vi "Photon Counter Control Panel (No Objects).vi"(8 "error in (no error)":errorcluster) -> (0 "error out":errorcluster)   [LabVIEW 2012]
uses:
  SR400/Public/Typedefs.llb/Gate Mode.ctl
  SR400/SR400.lvlib
panel:
  in  "VISA Resource Name":refnum<visa-resource-name>="GPIB0::23::INSTR"
  in  "Photon Counter SR 400":T1={"Mode"=0, "Count Time"=0.0, "Trigger Frequency"=10000000.0, "Trigger External?"=FALSE, "Gate A Mode"=0, "Gate A Width"=0.0, "Gate A Delay"=0.0, "Gate B Mode"=0, "Gate B Width"=0.0, "Gate B Delay"=0.0} {"Mode" items=["A,B For T Preset", "A-B For T Preset", "A+B For T Preset", "A For B Preset"]; "Gate A Mode" items=["CW", "Fixed"]; "Gate B Mode" items=["CW", "Fixed"]}
  out "Update visible/hidden":bool
  out "Gate B Mode":T2
  out "Gate A Mode":T2
  in  "stop":bool
  in  "Read to Control":bool
  in  "Read":bool
  in  "Initialize":bool
  out "Gate A % Current":dbl
  out "Gate B % Current":dbl
  in  "Gate B % Set":dbl
  in  "Gate A % Set":dbl
  in  "Gate Width: Time / Percent":bool caption="Gate Width\n        Time / Percent"
  in  "Gate Delay Reference\n        Start / Middle":bool
  in  "Gate B Mode Set":T2
  in  "Gate A Mode Set":T2
  out "Trigger Freq Current":dbl[unit]=42077.399999999994 caption="Trigger Freq"
  in  "Trigger Freq Set":dbl[unit]=42077.399999999994 caption="Trigger Freq."
  in  "Set Time & Freq.":bool
  in  "# Triggers vs Freq/Time":bool
  out "# of Cycles Current":dbl format="%^#_6g"
  in  "# of Cycles Set":dbl format="%^#_6g"
  in  "Set # of Triggers":bool
  in  "Internal / External":bool
  out "cpsB":dbl[unit] caption="CPS B"
  out "cpsA":dbl[unit] caption="CPS A"
  in  "Gate B Width Set":dbl[unit] caption="Gate B Width"
  in  "Gate A Width Set":dbl[unit]
  out "Gate A Width":dbl[unit] format="%^#_6g"
  out "Gate B Width":dbl[unit] format="%^#_6g"
  out "Gate B Delay":dbl[unit]
  out "Gate A Delay":dbl[unit]
  in  "Gate B Delay Set":dbl[unit]
  in  "Gate A Delay Set":dbl[unit]
  in  "Set Gate Delays":bool
  in  "Set Gate Mode":bool
  in  "Set Gate Widths":bool
  in  "Read Channels":bool
  in  "Count Time Set":dbl[unit]
  out "Count Time Current":dbl[unit]=1.0 min=0.0 max=10000.0 step=1.0 format="%#_7g"
  in  "Set Count Time":bool
  # "Gates"
  # "Trigger"
  # "Gate A"
  # "Gate B"
  # "Channels"
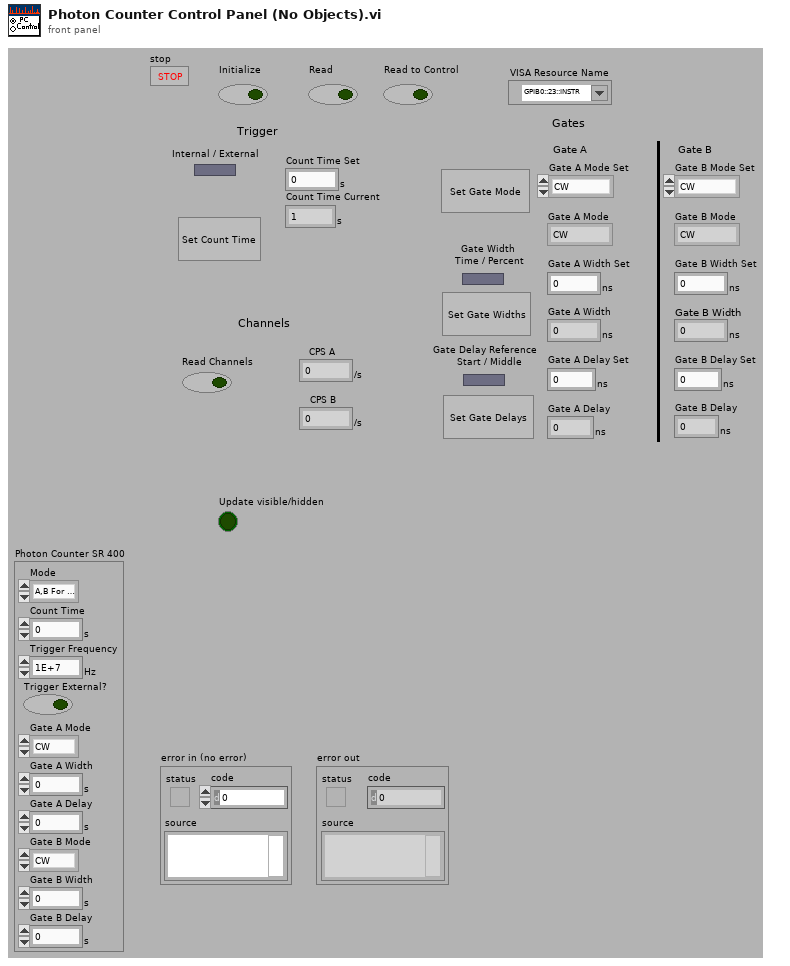
[diagram p1: front panel]
types:
  T1 = cluster{"Mode":u16, "Count Time":dbl[unit], "Trigger Frequency":dbl[unit], "Trigger External?":bool, "Gate A Mode":u16, "Gate A Width":dbl[unit], "Gate A Delay":dbl[unit], "Gate B Mode":u16, "Gate B Width":dbl[unit], "Gate B Delay":dbl[unit]}
  T2 = typedef "SR400.lvlib/Gate Mode.ctl" = enum16{"CW", "Fixed", "Scan"}
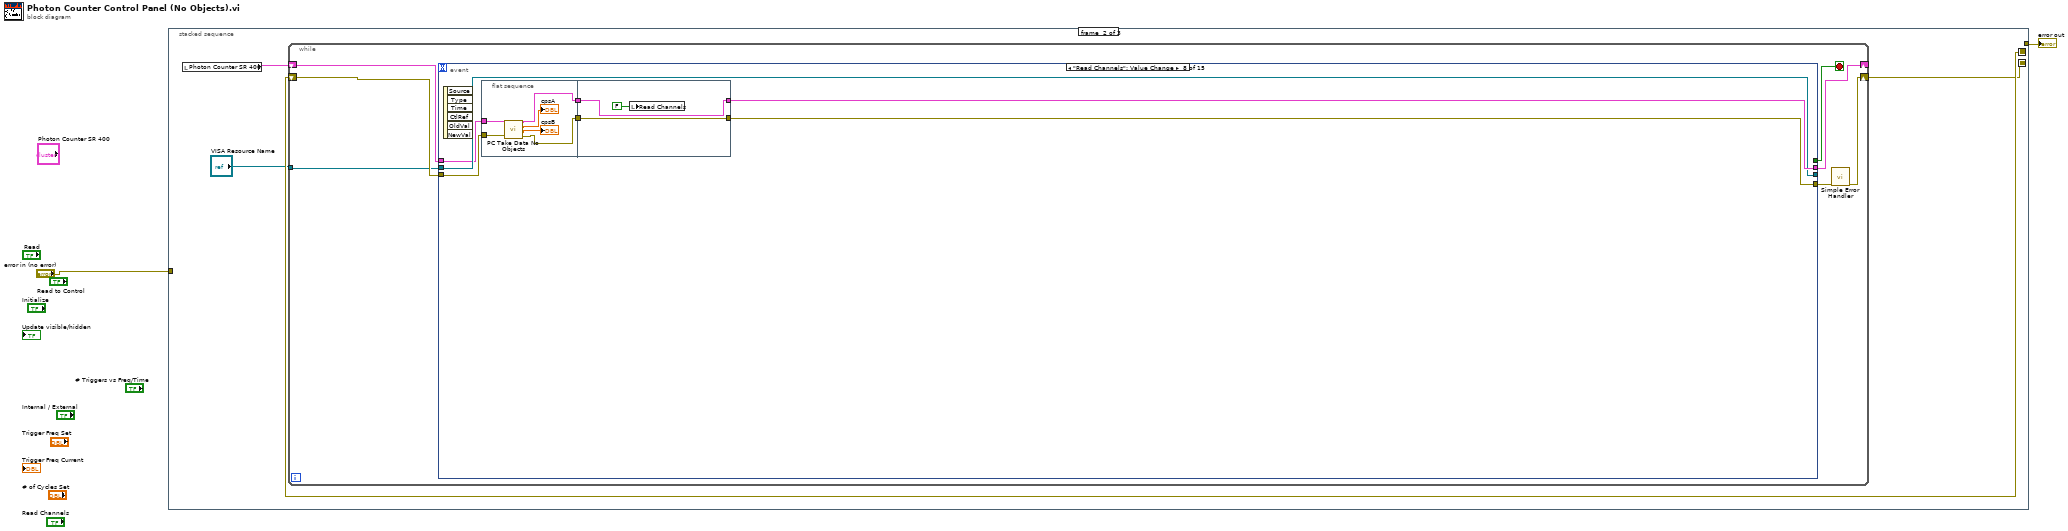
[diagram p0: block diagram]
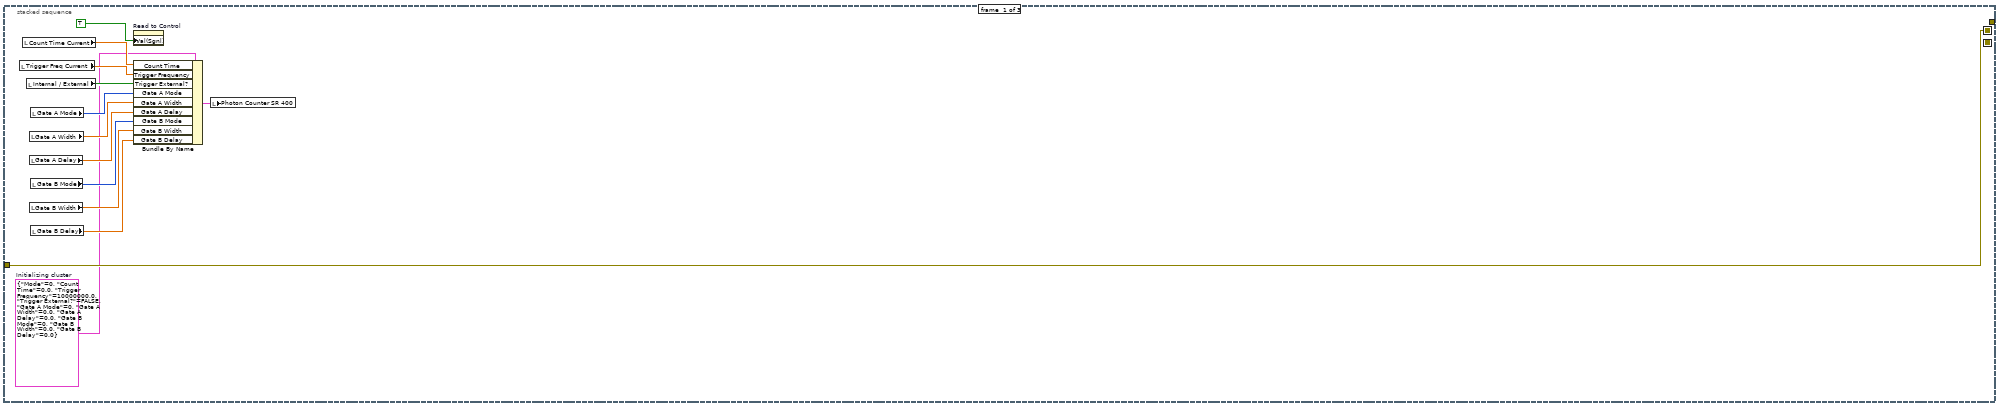
[diagram p2: hidden frame]
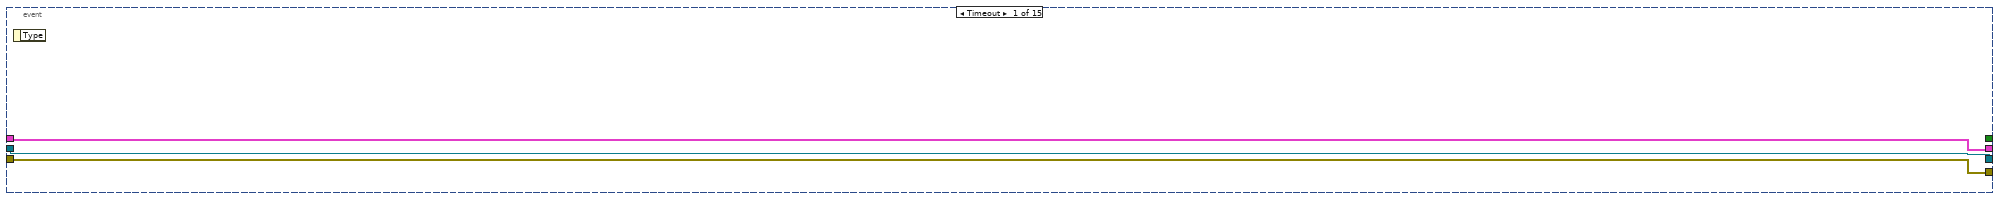
[diagram p3: hidden frame]
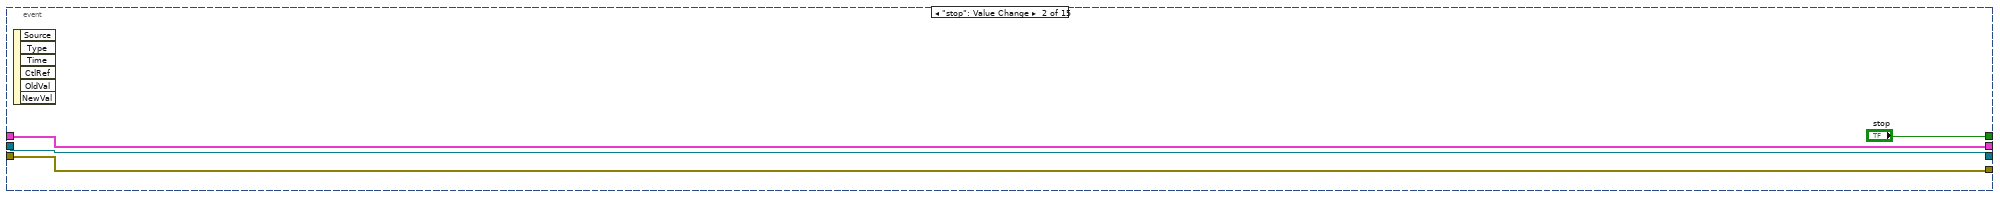
[diagram p4: hidden frame]
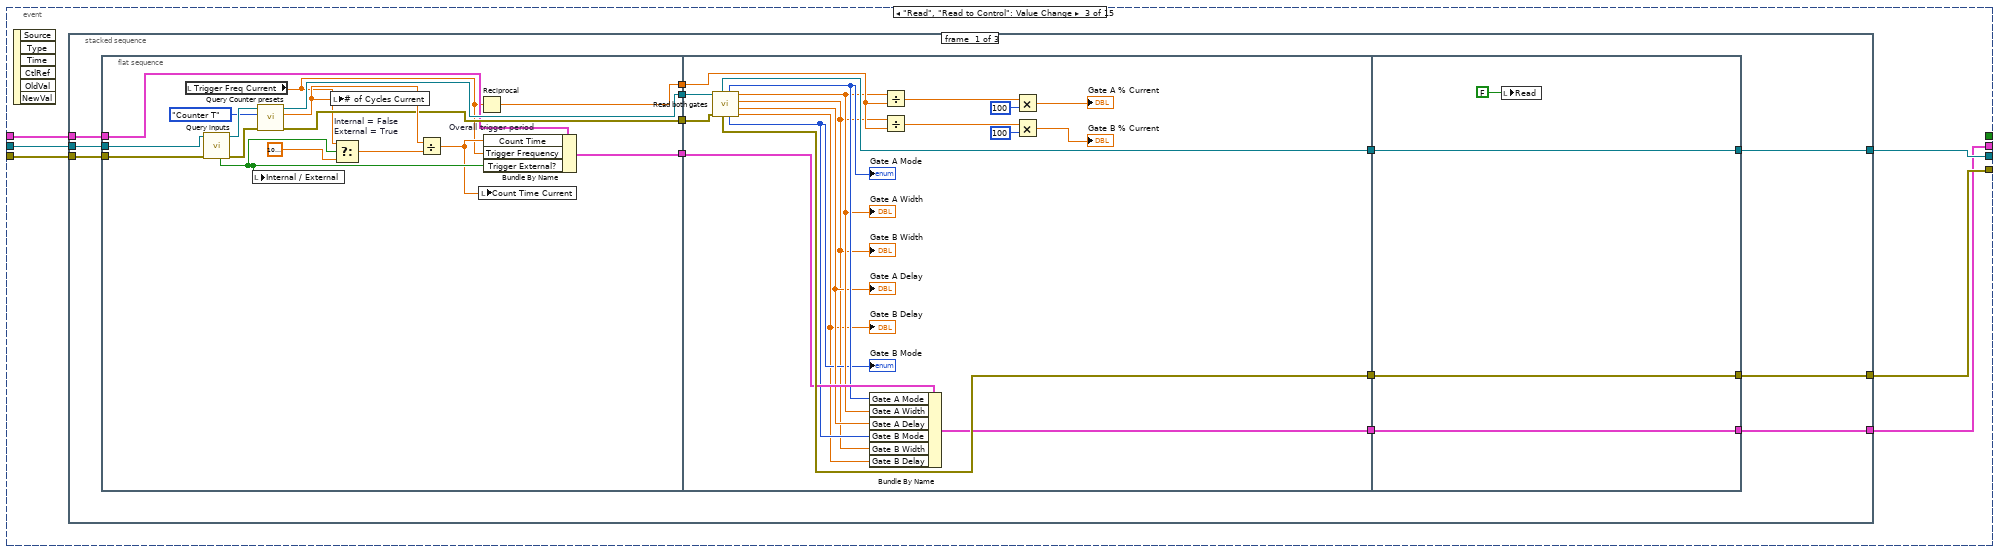
[diagram p5: hidden frame]
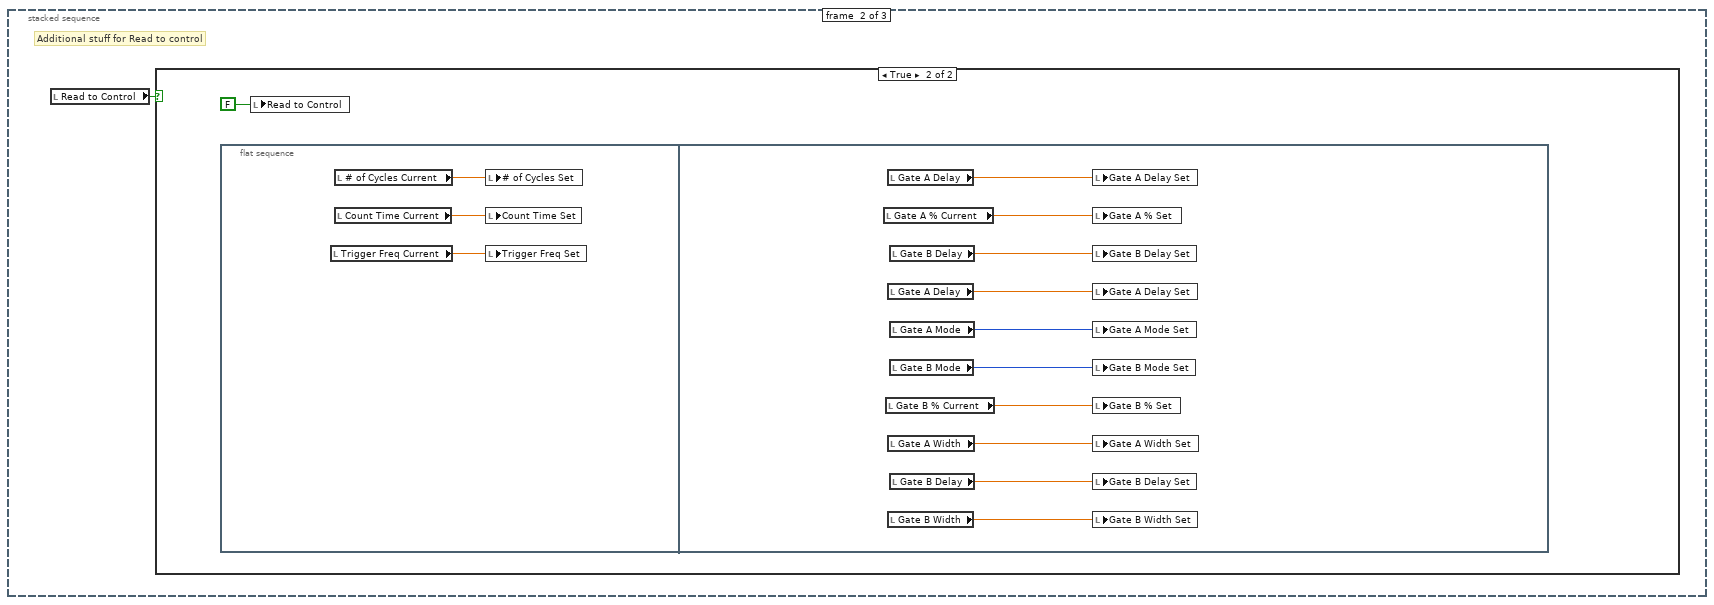
[diagram p6: hidden frame]
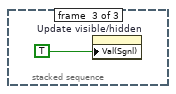
[diagram p8: hidden frame]
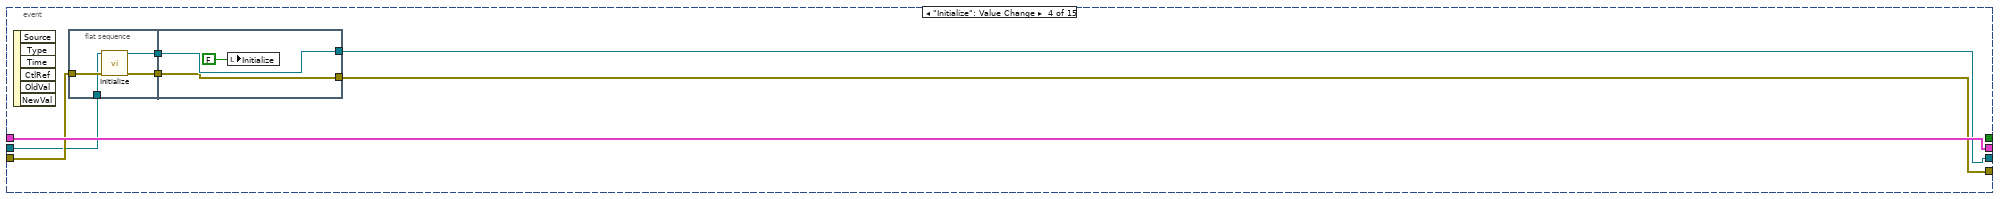
[diagram p9: hidden frame]
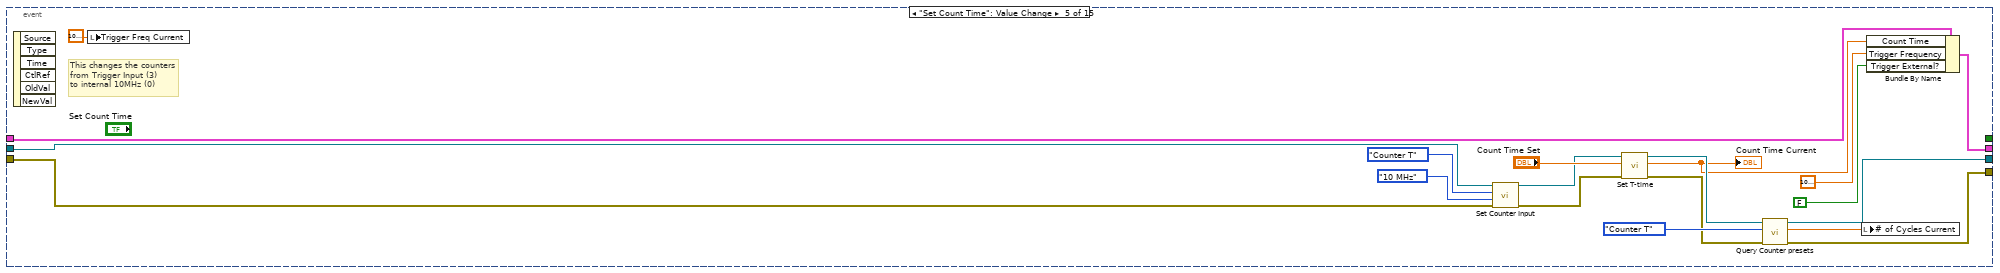
[diagram p10: hidden frame]
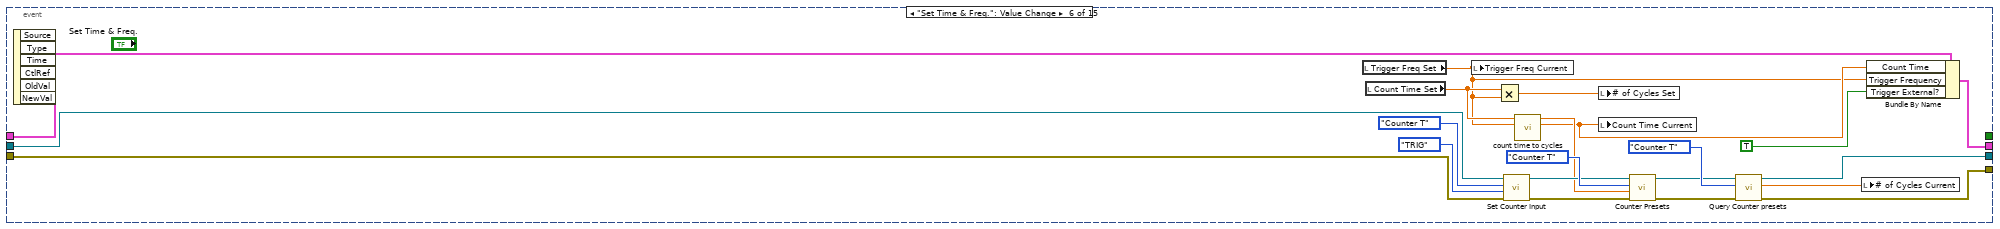
[diagram p11: hidden frame]
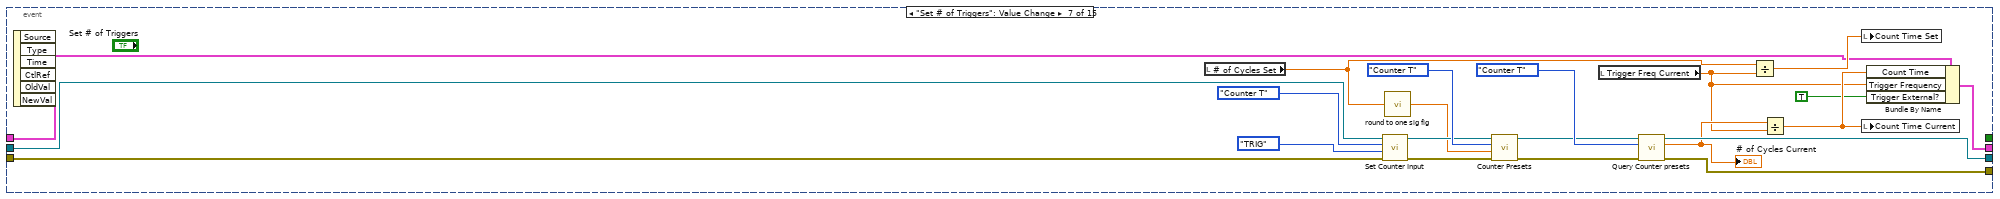
[diagram p12: hidden frame]
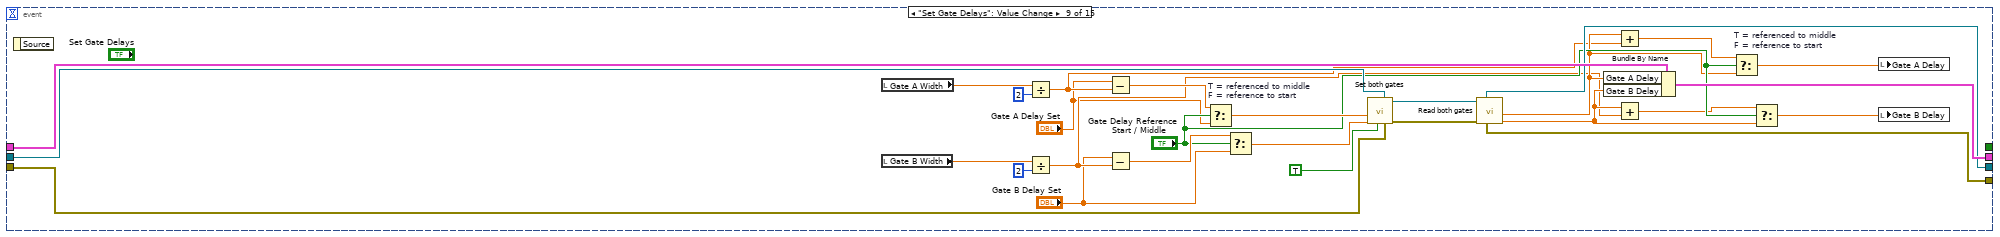
[diagram p13: hidden frame]
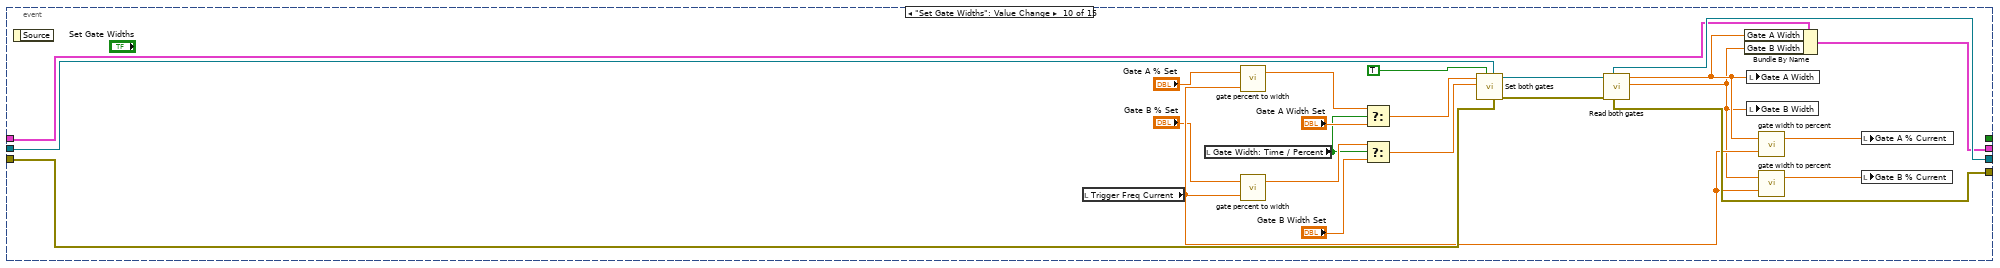
[diagram p14: hidden frame]
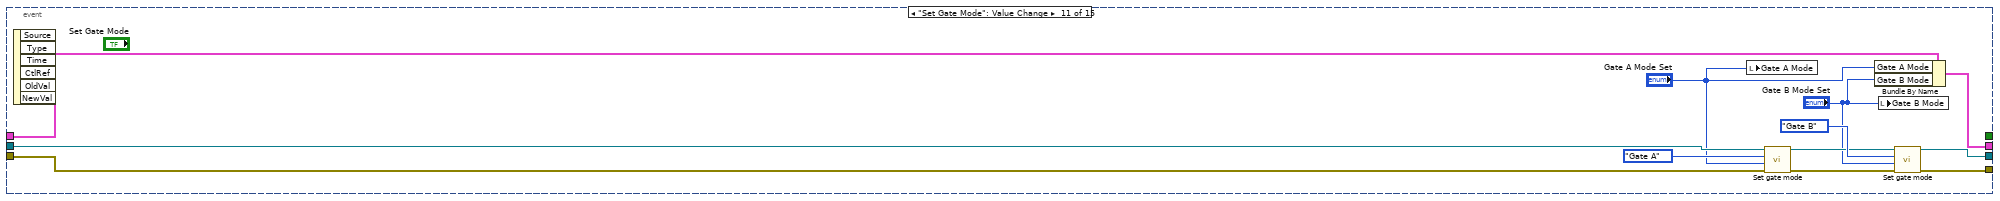
[diagram p15: hidden frame]
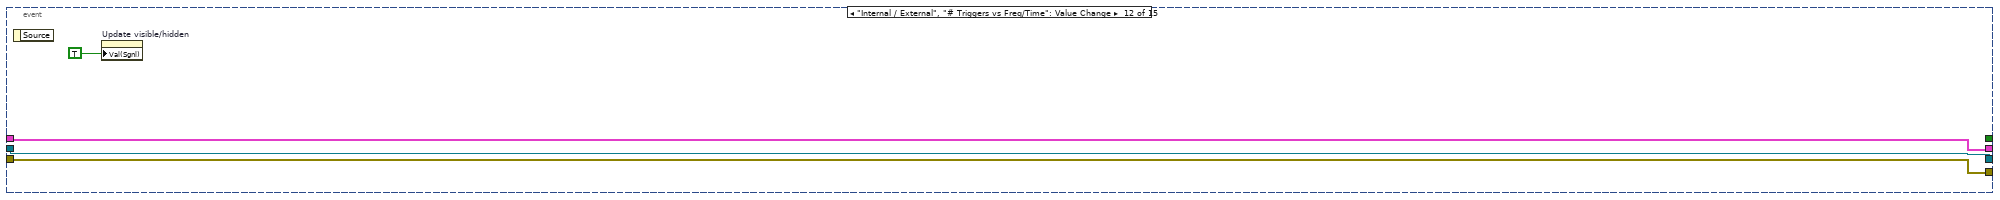
[diagram p16: hidden frame]
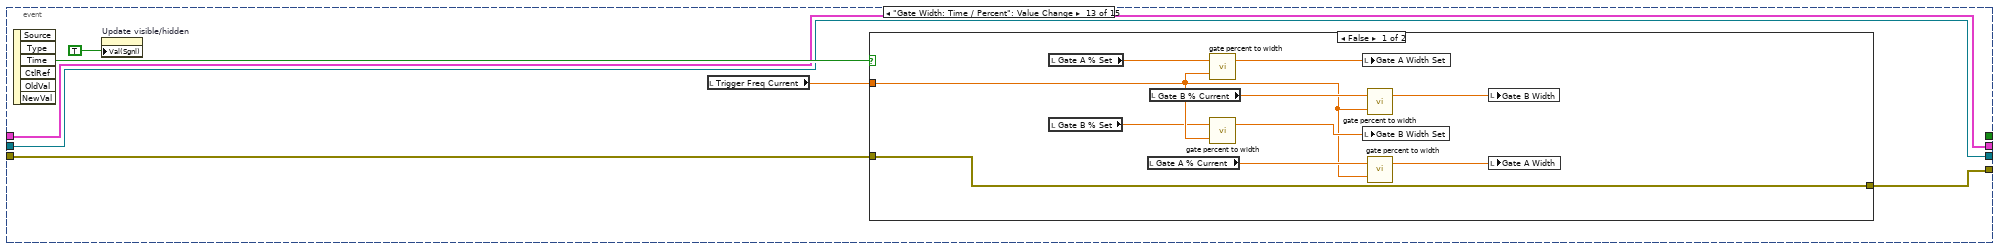
[diagram p17: hidden frame]
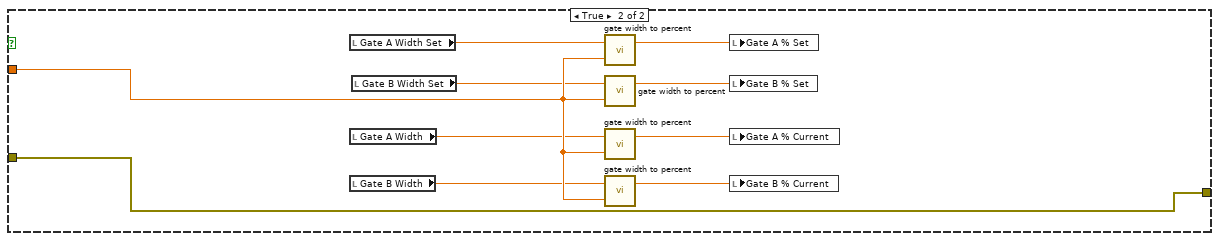
[diagram p18: hidden frame]
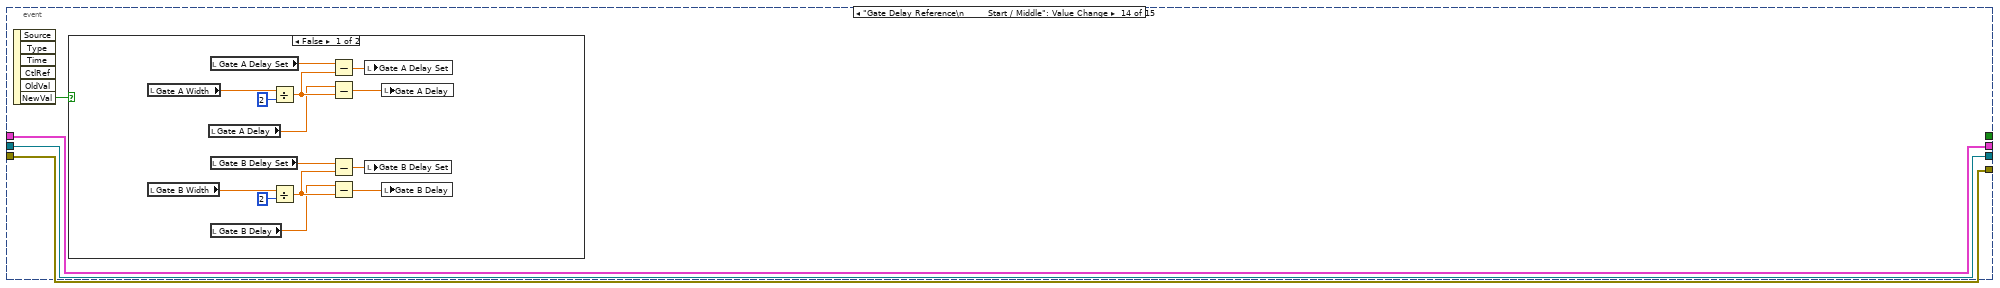
[diagram p19: hidden frame]
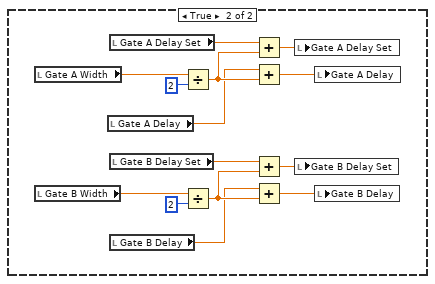
[diagram p20: hidden frame]
diagram:
  n1 = stacked-sequence {
    seq-local: [w5 _ _] -> [_ w19 _]
    seq-local: [_ w18 _] -> [_ _ w338]
    tunnel: "error in (no error)" -> [w5 _ _]
    tunnel: [_ _ w338] -> w2
    frame #0 {
      w3 = T1 {"Mode"=0, "Count Time"=0.0, "Trigger Frequency"=10000000.0, "Trigger External?"=FALSE, "Gate A Mode"=0, "Gate A Width"=0.0, "Gate A Delay"=0.0, "Gate B Mode"=0, "Gate B Width"=0.0, "Gate B Delay"=0.0}  # Initializing cluster
      n2 = local read "Trigger Freq Current"() -> (w13:dbl[unit])
      n3 = local read "Count Time Current"() -> (w14:dbl[unit])
      n4 = local read "Internal / External"() -> (w12:bool)
      n5 = local read "Gate A Width"() -> (w10:dbl[unit])
      n6 = local read "Gate A Delay"() -> (w9:dbl[unit])
      n7 = local read "Gate B Width"() -> (w7:dbl[unit])
      n8 = local read "Gate A Mode"() -> (w11:T2)
      n9 = local read "Gate B Mode"() -> (w6:T2)
      n10 = local read "Gate B Delay"() -> (w8:dbl[unit])
      n11 = property on="Read to Control" class="Bool (strict)"("Val(Sgnl)"=TRUE ("Value (Signaling)")) -> ()  [unwired: 2 in, 2 out]
      n12 = Bundle By Name(cluster=w3, "Count Time"=w14, "Trigger Frequency"=w13, "Trigger External?"=w12, "Gate A Mode"=w11, "Gate A Width"=w10, "Gate A Delay"=w9, "Gate B Mode"=w6, "Gate B Width"=w7, "Gate B Delay"=w8) -> (w4:T1)
      n13 = local write "Photon Counter SR 400"(w4) -> ()
    }
    frame #1 {
      n14 = local read "Photon Counter SR 400"() -> (w17:T1)
      n15 = while {
        shift-right: [w22] -> _
        shift-left: w17 -> [w21]
        shift-right: [w25] -> w18
        shift-left: w19 -> [w23]
        tunnel: "VISA Resource Name" -> [w20]
        stop <- w24 stop-if-true
        n16 = event shown="[7] \"Read Channels\": Value Change" {
          selector: _ -> [_ _ _ _ _ _ _ _ _ _ _ _ _ _ _]
          dyn-events: _ -> [_ _ _ _ _ _ _ _ _ _ _ _ _ _ _]
          timeout: _ -> [_ _ _ _ _ _ _ _ _ _ _ _ _ _ _]
          tunnel: [w28 w31 w37 w108 w137 w156 w180 w186 w212 w244 w254 w265 w268 w294 w327] -> _
          tunnel: w23 -> [w27 w30 w39 w113 w128 w150 w172 w189 w226 w245 w258 w264 w266 w293 w326]
          tunnel: [w27 w30 w36 w112 w136 w157 w179 w188 w210 w243 w255 w264 w267 w293 w326] -> w26
          tunnel: w20 -> [w28 w31 w38 w109 w129 w151 w173 w186 w225 w246 w259 w265 w268 w294 w327]
          tunnel: w21 -> [w29 w32 w35 w114 w126 w145 w166 w185 w224 w230 w253 w263 w269 w295 w325]
          tunnel: [w29 w32 w34 w114 w125 w144 w165 w187 w223 w229 w252 w263 w269 w295 w325] -> w22
          tunnel: [_ "stop" _ _ _ _ _ _ _ _ _ _ _ _ _] -> w24
          event Timeout {
            n17 = event-data() -> ()  [unwired: 2 out]
          }
          event "stop": Value Change {
            n18 = event-data() -> ()  [unwired: 7 out]
          }
          event "Read", "Read to Control": Value Change {
            n19 = event-data() -> ()  [unwired: 7 out]
            n20 = stacked-sequence {
              tunnel: w39 -> [w51 _ _]
              tunnel: w38 -> [w52 _ _]
              tunnel: [w47 _ _] -> w37
              tunnel: [w45 _ _] -> w36
              tunnel: w35 -> [w43 _ _]
              tunnel: [w41 _ _] -> w34
              frame #0 {
                n21 = flat-sequence {
                  tunnel: w52 -> [w68]
                  tunnel: w51 -> [w65]
                  tunnel: [w61] -> w50
                  tunnel: [w60] -> w49
                  tunnel: [w59] -> w48
                  tunnel: w43 -> [w57]
                  tunnel: [w53] -> w42
                  tunnel: w50 -> [w81]
                  tunnel: w49 -> [w80]
                  tunnel: w48 -> [w79]
                  tunnel: [w78] -> w46
                  tunnel: [w77] -> w44
                  tunnel: w42 -> [w76]
                  tunnel: [w69] -> w40
                  tunnel: [w90] -> w47
                  tunnel: w46 -> [w90]
                  tunnel: [w89] -> w45
                  tunnel: w44 -> [w89]
                  tunnel: [w88] -> w41
                  tunnel: w40 -> [w88]
                  frame #0 {
                    n22 = local read "Trigger Freq Current"() -> (w54:dbl[unit])
                    n23 = call "Query inputs.vi"("error in (no error)"=w65, "VISA resource name"=w68) -> ("error out"=w66:errorcluster, "VISA resource name out"=w67:refnum<visa-resource-name>, "Externally-triggered?"=w56:bool)  [unwired: 7 out]
                    n24 = local write "Internal / External"(w56) -> ()
                    n25 = call "Query Counter presets.vi"("error in (no error)"=w66, "Counter (Def: T)"=enum16{"Invalid", "Counter B", "Counter T"}."Counter T" ("i (0)"), "VISA resource name"=w67) -> ("error out"=w60:errorcluster, "Number of triggers"=w62:dbl, "VISA resource name out"=w61:refnum<visa-resource-name>)  [unwired: 6 out]
                    n26 = local write "# of Cycles Current"(w62) -> ()
                    n27 = Select "Internal = False\nExternal = True"(t=w54, s=w56, f=dbl[unit] 10000000.0 ("freq")) -> (s? t:f=w63:dbl[unit])
                    n28 = Divide(x=w62, y=w63) -> (x/y=w55:dbl[unit])
                    n29 = Reciprocal "Overall trigger period"(x=w54) -> (1/x=w59:dbl[unit])
                    n30 = local write "Count Time Current"(w55) -> ()
                    n31 = Bundle By Name(cluster=w57, "Count Time"=w55, "Trigger Frequency"=w54, "Trigger External?"=w56) -> (w53:T1)
                  }
                  frame #1 {
                    n32 = call "Read both gates.vi"("error in (no error)"=w80, "VISA resource name"=w81) -> ("Gate B Delay"=w70:dbl[unit], "Gate A Delay"=w73:dbl[unit], "Gate B Width"=w71:dbl[unit], "Gate A Width"=w74:dbl[unit], "Current mode B"=w72:enum16{"CW", "Fixed", "Scan"}, "Current mode A"=w75:enum16{"CW", "Fixed", "Scan"}, "error out"=w77:errorcluster, "VISA resource name out"=w78:refnum<visa-resource-name>)  [unwired: 2 out]
                    "Gate B Width" <- w71
                    "Gate A Width" <- w74
                    "Gate A Delay" <- w73
                    "Gate B Delay" <- w70
                    "Gate A Mode" <- w75
                    "Gate B Mode" <- w72
                    n33 = Bundle By Name(cluster=w76, "Gate A Mode"=w75, "Gate A Width"=w74, "Gate A Delay"=w73, "Gate B Mode"=w72, "Gate B Width"=w71, "Gate B Delay"=w70) -> (w69:T1)
                    n34 = Divide(x=w74, y=w79) -> (x/y=w83:dbl)
                    n35 = Divide(x=w71, y=w79) -> (x/y=w85:dbl)
                    n36 = Multiply(x=w83, y=i8 100) -> (x*y=→"Gate A % Current":dbl)
                    n37 = Multiply(x=w85, y=i8 100) -> (x*y=→"Gate B % Current":dbl)
                  }
                  frame #2 {
                    n38 = local write "Read"(FALSE ("Read")) -> ()
                  }
                }
              }
              frame #1 {
                # "Additional stuff for Read to control"
                n39 = local read "Read to Control"() -> (w92:bool)
                n40 = case shown="True" w92 {
                  frame False {
                  }
                  frame True {
                    n41 = flat-sequence {
                      frame #0 {
                        n42 = local read "Trigger Freq Current"() -> (w94:dbl[unit])
                        n43 = local read "# of Cycles Current"() -> (w95:dbl)
                        n44 = local read "Count Time Current"() -> (w96:dbl[unit])
                        n45 = local write "# of Cycles Set"(w95) -> ()
                        n46 = local write "Count Time Set"(w96) -> ()
                        n47 = local write "Trigger Freq Set"(w94) -> ()
                      }
                      frame #1 {
                        n48 = local read "Gate A % Current"() -> (w103:dbl)
                        n49 = local read "Gate B % Current"() -> (w105:dbl)
                        n50 = local read "Gate A Delay"() -> (w98:dbl[unit])
                        n51 = local read "Gate A Delay"() -> (w104:dbl[unit])
                        n52 = local read "Gate A Width"() -> (w102:dbl[unit])
                        n53 = local read "Gate B Width"() -> (w97:dbl[unit])
                        n54 = local read "Gate B Delay"() -> (w99:dbl[unit])
                        n55 = local read "Gate A Mode"() -> (w100:T2)
                        n56 = local read "Gate B Mode"() -> (w101:T2)
                        n57 = local read "Gate B Delay"() -> (w106:dbl[unit])
                        n58 = local write "Gate A Delay Set"(w98) -> ()
                        n59 = local write "Gate A % Set"(w103) -> ()
                        n60 = local write "Gate B Delay Set"(w99) -> ()
                        n61 = local write "Gate A Delay Set"(w104) -> ()
                        n62 = local write "Gate A Mode Set"(w100) -> ()
                        n63 = local write "Gate B Mode Set"(w101) -> ()
                        n64 = local write "Gate B % Set"(w105) -> ()
                        n65 = local write "Gate A Width Set"(w102) -> ()
                        n66 = local write "Gate B Delay Set"(w106) -> ()
                        n67 = local write "Gate B Width Set"(w97) -> ()
                      }
                    }
                    n68 = local write "Read to Control"(FALSE ("Read to Control")) -> ()
                  }
                }
              }
              frame #2 {
                n69 = property on="Update visible/hidden" class="Bool (strict)"("Val(Sgnl)"=TRUE ("Value (Signaling)")) -> ()  [unwired: 2 in, 2 out]
              }
            }
          }
          event "Initialize": Value Change {
            n70 = event-data() -> ()  [unwired: 7 out]
            n71 = flat-sequence {
              tunnel: w113 -> [w118]
              tunnel: [w117] -> w111
              tunnel: [w116] -> w110
              tunnel: w109 -> [w115]
              tunnel: [w120] -> w112
              tunnel: [w121] -> w108
              tunnel: w111 -> [w121]
              tunnel: w110 -> [w120]
              frame #0 {
                n72 = call "Initialize.vi"("errorIN"=w118, "VISA resource name"=w115) -> ("errorOUT"=w116:errorcluster, "VISA resource name out"=w117:refnum<visa-resource-name>)  [unwired: 8 out]
              }
              frame #1 {
                n73 = local write "Initialize"(FALSE ("Re-initialize")) -> ()
              }
            }
          }
          event "Set Count Time": Value Change {
            # "This changes the counters\nfrom Trigger Input (3)\nto internal 10MHz (0)"
            n74 = event-data() -> ()  [unwired: 7 out]
            n75 = local write "Trigger Freq Current"(dbl[unit] 10000000.0 ("freq")) -> ()
            n76 = call "Set Counter Input.vi"("error in (no error)"=w128, "Input (def: 10 MHz)"=enum16{"10 MHz", "INPUT 1", "INPUT 2", "TRIG"}."10 MHz" ("n (0.000000)"), "Counter (def: A)"=enum16{"Counter A", "Counter B", "Counter T"}."Counter T" ("i (0) 2"), "VISA resource name"=w129) -> ("error out"=w131:errorcluster, "VISA resource name out"=w130:refnum<visa-resource-name>)  [unwired: 6 out]
            n77 = call "Set T-time.vi"("errorIN"=w131, "Count Time Set"="Count Time Set", "VISA resource name"=w130) -> ("errorOUT"=w132:errorcluster, "ttimeOUT"=w124:dbl[unit], "VISA resource name out"=w135:refnum<visa-resource-name>)  [unwired: 4 out]
            "Count Time Current" <- w124
            n78 = call "Query Counter presets.vi"("error in (no error)"=w132, "Counter (Def: T)"=enum16{"Invalid", "Counter B", "Counter T"}."Counter T" ("i (0)"), "VISA resource name"=w135) -> ("error out"=w136:errorcluster, "Number of triggers"=w138:dbl, "VISA resource name out"=w137:refnum<visa-resource-name>)  [unwired: 6 out]
            n79 = local write "# of Cycles Current"(w138) -> ()
            n80 = Bundle By Name(cluster=w126, "Count Time"=w124, "Trigger Frequency"=dbl[unit] 10000000.0, "Trigger External?"=FALSE) -> (w125:T1)
          }
          event "Set Time & Freq.": Value Change {
            n81 = event-data() -> ()  [unwired: 7 out]
            n82 = local read "Trigger Freq Set"() -> (w141:dbl[unit])
            n83 = local read "Count Time Set"() -> (w146:dbl[unit])
            n84 = local write "Trigger Freq Current"(w141) -> ()
            n85 = Multiply(x=w146, y=w141) -> (x*y=w147:dbl)
            n86 = call "Set Counter Input.vi"("error in (no error)"=w150, "Input (def: 10 MHz)"=enum16{"10 MHz", "INPUT 1", "INPUT 2", "TRIG"}."TRIG" ("n (0.000000)"), "Counter (def: A)"=enum16{"Counter A", "Counter B", "Counter T"}."Counter T" ("i (0) 2"), "VISA resource name"=w151) -> ("error out"=w152:errorcluster, "VISA resource name out"=w153:refnum<visa-resource-name>)  [unwired: 6 out]
            n87 = call "count time to cycles.vi"("Trigger Freq"=w141, "Count Time Set"=w146) -> ("Count Time Current"=w142:dbl[unit], "Number of triggers"=w148:dbl)  [unwired: 1 in, 3 out]
            n88 = local write "# of Cycles Set"(w147) -> ()
            n89 = local write "Count Time Current"(w142) -> ()
            n90 = call "Counter Presets.vi"("error in (no error)"=w152, "Number of triggers"=w148, "Counter (Def: T)"=enum16{"Invalid", "Counter B", "Counter T"}."Counter T" ("i (0) 2"), "VISA resource name"=w153) -> ("error out"=w158:errorcluster, "VISA resource name out"=w155:refnum<visa-resource-name>)  [unwired: 6 out]
            n91 = call "Query Counter presets.vi"("error in (no error)"=w158, "Counter (Def: T)"=enum16{"Invalid", "Counter B", "Counter T"}."Counter T" ("i (0)"), "VISA resource name"=w155) -> ("error out"=w157:errorcluster, "Number of triggers"=w159:dbl, "VISA resource name out"=w156:refnum<visa-resource-name>)  [unwired: 6 out]
            n92 = local write "# of Cycles Current"(w159) -> ()
            n93 = Bundle By Name(cluster=w145, "Count Time"=w142, "Trigger Frequency"=w141, "Trigger External?"=TRUE) -> (w144:T1)
          }
          event "Set # of Triggers": Value Change {
            n94 = event-data() -> ()  [unwired: 7 out]
            n95 = local read "# of Cycles Set"() -> (w170:dbl)
            n96 = call "Set Counter Input.vi"("error in (no error)"=w172, "Input (def: 10 MHz)"=enum16{"10 MHz", "INPUT 1", "INPUT 2", "TRIG"}."TRIG" ("n (0.000000)"), "Counter (def: A)"=enum16{"Counter A", "Counter B", "Counter T"}."Counter T" ("i (0) 2"), "VISA resource name"=w173) -> ("error out"=w174:errorcluster, "VISA resource name out"=w175:refnum<visa-resource-name>)  [unwired: 6 out]
            n97 = call "round to one sig fig.vi"("input number"=w170) -> ("rounded to 1 sig fig"=w168:dbl)
            n98 = call "Counter Presets.vi"("error in (no error)"=w174, "Number of triggers"=w168, "Counter (Def: T)"=enum16{"Invalid", "Counter B", "Counter T"}."Counter T" ("i (0) 2"), "VISA resource name"=w175) -> ("error out"=w178:errorcluster, "VISA resource name out"=w177:refnum<visa-resource-name>)  [unwired: 6 out]
            n99 = local read "Trigger Freq Current"() -> (w162:dbl[unit])
            n100 = call "Query Counter presets.vi"("error in (no error)"=w178, "Counter (Def: T)"=enum16{"Invalid", "Counter B", "Counter T"}."Counter T" ("i (0)"), "VISA resource name"=w177) -> ("error out"=w179:errorcluster, "Number of triggers"=w167:dbl, "VISA resource name out"=w180:refnum<visa-resource-name>)  [unwired: 6 out]
            "# of Cycles Current" <- w167
            n101 = Divide(x=w170, y=w162) -> (x/y=w169:dbl[unit])
            n102 = Divide(x=w167, y=w162) -> (x/y=w164:dbl[unit])
            n103 = local write "Count Time Set"(w169) -> ()
            n104 = local write "Count Time Current"(w164) -> ()
            n105 = Bundle By Name(cluster=w166, "Count Time"=w164, "Trigger Frequency"=w162, "Trigger External?"=TRUE) -> (w165:T1)
          }
          event "Read Channels": Value Change {
            n106 = event-data() -> ()  [unwired: 7 out]
            n107 = flat-sequence {
              tunnel: w189 -> [w195]
              tunnel: w185 -> [w191]
              tunnel: [w194] -> w184
              tunnel: [w190] -> w183
              tunnel: [w197] -> w187
              tunnel: [w198] -> w188
              tunnel: w184 -> [w198]
              tunnel: w183 -> [w197]
              frame #0 {
                n108 = call "PC Take Data No Objects.vi"("error in (no error)"=w195, "Photon Counter SR 400 in"=w191) -> ("error out"=w194:errorcluster, "CPS B"=→"cpsB":dbl[unit], "CPS A"=→"cpsA":dbl[unit], "Photon counter SR 400 out"=w190:T1)  [unwired: 6 in]
              }
              frame #1 {
                n109 = local write "Read Channels"(FALSE ("Read Channels")) -> ()
              }
            }
          }
          event "Set Gate Delays": Value Change {
            n110 = event-data() -> ()  [unwired: 2 out]
            n111 = local read "Gate A Width"() -> (w221:dbl[unit])
            n112 = local read "Gate B Width"() -> (w220:dbl[unit])
            n113 = Divide(x=w221, y=2) -> (x/y=w200:dbl[unit])
            n114 = Divide(x=w220, y=2) -> (x/y=w202:dbl[unit])
            n115 = Subtract(x="Gate A Delay Set", y=w200) -> (x-y=w217:dbl[unit])
            n116 = Subtract(x="Gate B Delay Set", y=w202) -> (x-y=w215:dbl[unit])
            n117 = Select "T = referenced to middle\nF = reference to start"(t=w217, s="Gate Delay Reference\n        Start / Middle", f="Gate A Delay Set") -> (s? t:f=w214:dbl[unit])
            n118 = Select(t=w215, s="Gate Delay Reference\n        Start / Middle", f="Gate B Delay Set") -> (s? t:f=w216:dbl[unit])
            n119 = call "Set both gates.vi"("Error In"=w226, "VISA resource name"=w225, "Set Delay?"=TRUE, "gatedelayoffsetB"=w216, "gatedelayoffsetA"=w214) -> ("Error Out"=w211:errorcluster, "VISA resource name out"=w213:refnum<visa-resource-name>)  [unwired: 3 in, 2 out]
            n120 = call "Read both gates.vi"("error in (no error)"=w211, "VISA resource name"=w213) -> ("Gate B Delay"=w207:dbl[unit], "Gate A Delay"=w208:dbl[unit], "error out"=w210:errorcluster, "VISA resource name out"=w212:refnum<visa-resource-name>)  [unwired: 6 out]
            n121 = Bundle By Name(cluster=w224, "Gate A Delay"=w208, "Gate B Delay"=w207) -> (w223:T1)
            n122 = Add(x=w208, y=w200) -> (x+y=w206:dbl[unit])
            n123 = Add(x=w207, y=w202) -> (x+y=w205:dbl[unit])
            n124 = Select "T = referenced to middle\nF = reference to start"(t=w206, s="Gate Delay Reference\n        Start / Middle", f=w208) -> (s? t:f=w204:dbl[unit])
            n125 = Select(t=w205, s="Gate Delay Reference\n        Start / Middle", f=w207) -> (s? t:f=w203:dbl[unit])
            n126 = local write "Gate A Delay"(w204) -> ()
            n127 = local write "Gate B Delay"(w203) -> ()
          }
          event "Set Gate Widths": Value Change {
            n128 = event-data() -> ()  [unwired: 2 out]
            n129 = local read "Trigger Freq Current"() -> (w240:dbl[unit])
            n130 = local read "Gate Width: Time / Percent"() -> (w233:bool)
            n131 = call "gate percent to width.vi"("Trigger Freq"=w240, "Gate %"="Gate A % Set") -> ("Gate width"=w235:dbl[unit])  [unwired: 1 out]
            n132 = call "gate percent to width.vi"("Trigger Freq"=w240, "Gate %"="Gate B % Set") -> ("Gate width"=w234:dbl[unit])  [unwired: 1 out]
            n133 = Select(t=w235, s=w233, f="Gate A Width Set") -> (s? t:f=w236:dbl[unit])
            n134 = Select(t=w234, s=w233, f="Gate B Width Set") -> (s? t:f=w231:dbl[unit])
            n135 = call "Set both gates.vi"("Error In"=w245, "VISA resource name"=w246, "Set Width?"=TRUE, "Gate B Width"=w231, "Gate A Width"=w236) -> ("Error Out"=w249:errorcluster, "VISA resource name out"=w248:refnum<visa-resource-name>)  [unwired: 3 in, 2 out]
            n136 = call "Read both gates.vi"("error in (no error)"=w249, "VISA resource name"=w248) -> ("Gate B Width"=w227:dbl[unit], "Gate A Width"=w228:dbl[unit], "error out"=w243:errorcluster, "VISA resource name out"=w244:refnum<visa-resource-name>)  [unwired: 6 out]
            n137 = Bundle By Name(cluster=w230, "Gate A Width"=w228, "Gate B Width"=w227) -> (w229:T1)
            n138 = local write "Gate A Width"(w228) -> ()
            n139 = local write "Gate B Width"(w227) -> ()
            n140 = call "gate width to percent.vi"("Trigger Freq"=w240, "Gate width"=w228) -> ("Gate %"=w241:dbl)  [unwired: 1 out]
            n141 = call "gate width to percent.vi"("Trigger Freq"=w240, "Gate width"=w227) -> ("Gate %"=w242:dbl)  [unwired: 1 out]
            n142 = local write "Gate A % Current"(w241) -> ()
            n143 = local write "Gate B % Current"(w242) -> ()
          }
          event "Set Gate Mode": Value Change {
            n144 = event-data() -> ()  [unwired: 7 out]
            n145 = local write "Gate A Mode"("Gate A Mode Set") -> ()
            n146 = call "Set gate mode.vi"("error in (no error)"=w258, "Mode (def: CW)"="Gate A Mode Set", "Gate (def: A)"=enum16{"Gate A", "Gate B"}."Gate A" ("i (0)"), "VISA resource name"=w259) -> ("error out"=w257:errorcluster, "VISA resource name out"=w256:refnum<visa-resource-name>)  [unwired: 6 out]
            n147 = Bundle By Name(cluster=w253, "Gate A Mode"="Gate A Mode Set", "Gate B Mode"="Gate B Mode Set") -> (w252:T1)
            n148 = local write "Gate B Mode"("Gate B Mode Set") -> ()
            n149 = call "Set gate mode.vi"("error in (no error)"=w257, "Mode (def: CW)"="Gate B Mode Set", "Gate (def: A)"=enum16{"Gate A", "Gate B"}."Gate B" ("i (0)"), "VISA resource name"=w256) -> ("error out"=w255:errorcluster, "VISA resource name out"=w254:refnum<visa-resource-name>)  [unwired: 6 out]
          }
          event "Internal / External", "# Triggers vs Freq/Time": Value Change {
            n150 = event-data() -> ()  [unwired: 2 out]
            n151 = property on="Update visible/hidden" class="Bool (strict)"("Val(Sgnl)"=TRUE ("Value (Signaling)")) -> ()  [unwired: 2 in, 2 out]
          }
          event "Gate Width: Time / Percent": Value Change {
            n152 = event-data() -> ("NewVal"=w270:bool)  [unwired: 6 out]
            n153 = property on="Update visible/hidden" class="Bool (strict)"("Val(Sgnl)"=TRUE ("Value (Signaling)")) -> ()  [unwired: 2 in, 2 out]
            n154 = local read "Trigger Freq Current"() -> (w271:dbl[unit])
            n155 = case shown="False" w270 {
              tunnel: w271 -> [w276 w292]
              tunnel: [w273 w283] -> w267
              tunnel: w266 -> [w273 w283]
              frame False {
                n156 = local read "Gate A % Set"() -> (w274:dbl)
                n157 = local read "Gate B % Set"() -> (w275:dbl)
                n158 = local read "Gate A % Current"() -> (w280:dbl)
                n159 = local read "Gate B % Current"() -> (w279:dbl)
                n160 = call "gate percent to width.vi"("Trigger Freq"=w276, "Gate %"=w274) -> ("Gate width"=w282:dbl[unit])  [unwired: 1 out]
                n161 = call "gate percent to width.vi"("Trigger Freq"=w276, "Gate %"=w275) -> ("Gate width"=w281:dbl[unit])  [unwired: 1 out]
                n162 = local write "Gate A Width Set"(w282) -> ()
                n163 = local write "Gate B Width Set"(w281) -> ()
                n164 = call "gate percent to width.vi"("Trigger Freq"=w276, "Gate %"=w279) -> ("Gate width"=w277:dbl[unit])  [unwired: 1 out]
                n165 = call "gate percent to width.vi"("Trigger Freq"=w276, "Gate %"=w280) -> ("Gate width"=w278:dbl[unit])  [unwired: 1 out]
                n166 = local write "Gate B Width"(w277) -> ()
                n167 = local write "Gate A Width"(w278) -> ()
              }
              frame True {
                n168 = local read "Gate A Width Set"() -> (w291:dbl[unit])
                n169 = local read "Gate A Width"() -> (w287:dbl[unit])
                n170 = local read "Gate B Width"() -> (w285:dbl[unit])
                n171 = local read "Gate B Width Set"() -> (w289:dbl[unit])
                n172 = call "gate width to percent.vi"("Trigger Freq"=w292, "Gate width"=w291) -> ("Gate %"=w290:dbl)  [unwired: 1 out]
                n173 = call "gate width to percent.vi"("Trigger Freq"=w292, "Gate width"=w289) -> ("Gate %"=w288:dbl)  [unwired: 1 out]
                n174 = call "gate width to percent.vi"("Trigger Freq"=w292, "Gate width"=w287) -> ("Gate %"=w286:dbl)  [unwired: 1 out]
                n175 = call "gate width to percent.vi"("Trigger Freq"=w292, "Gate width"=w285) -> ("Gate %"=w284:dbl)  [unwired: 1 out]
                n176 = local write "Gate A % Set"(w290) -> ()
                n177 = local write "Gate B % Set"(w288) -> ()
                n178 = local write "Gate A % Current"(w286) -> ()
                n179 = local write "Gate B % Current"(w284) -> ()
              }
            }
          }
          event "Gate Delay Reference\n        Start / Middle": Value Change {
            n180 = event-data() -> ("NewVal"=w296:bool)  [unwired: 6 out]
            n181 = case shown="False" w296 {
              frame False {
                n182 = local read "Gate A Width"() -> (w310:dbl[unit])
                n183 = local read "Gate B Width"() -> (w307:dbl[unit])
                n184 = local read "Gate A Delay"() -> (w303:dbl[unit])
                n185 = local read "Gate A Delay Set"() -> (w305:dbl[unit])
                n186 = local read "Gate B Delay Set"() -> (w300:dbl[unit])
                n187 = local read "Gate B Delay"() -> (w298:dbl[unit])
                n188 = Divide(x=w310, y=2) -> (x/y=w306:dbl[unit])
                n189 = Divide(x=w307, y=2) -> (x/y=w301:dbl[unit])
                n190 = Subtract(x=w305, y=w306) -> (x-y=w304:dbl[unit])
                n191 = Subtract(x=w303, y=w306) -> (x-y=w302:dbl[unit])
                n192 = Subtract(x=w300, y=w301) -> (x-y=w299:dbl[unit])
                n193 = Subtract(x=w298, y=w301) -> (x-y=w297:dbl[unit])
                n194 = local write "Gate A Delay Set"(w304) -> ()
                n195 = local write "Gate B Delay Set"(w299) -> ()
                n196 = local write "Gate A Delay"(w302) -> ()
                n197 = local write "Gate B Delay"(w297) -> ()
              }
              frame True {
                n198 = local read "Gate A Width"() -> (w324:dbl[unit])
                n199 = local read "Gate B Width"() -> (w321:dbl[unit])
                n200 = local read "Gate A Delay"() -> (w317:dbl[unit])
                n201 = local read "Gate A Delay Set"() -> (w319:dbl[unit])
                n202 = local read "Gate B Delay Set"() -> (w314:dbl[unit])
                n203 = local read "Gate B Delay"() -> (w312:dbl[unit])
                n204 = Divide(x=w324, y=2) -> (x/y=w320:dbl[unit])
                n205 = Divide(x=w321, y=2) -> (x/y=w315:dbl[unit])
                n206 = Add(x=w319, y=w320) -> (x+y=w318:dbl[unit])
                n207 = Add(x=w317, y=w320) -> (x+y=w316:dbl[unit])
                n208 = Add(x=w314, y=w315) -> (x+y=w313:dbl[unit])
                n209 = Add(x=w312, y=w315) -> (x+y=w311:dbl[unit])
                n210 = local write "Gate A Delay Set"(w318) -> ()
                n211 = local write "Gate B Delay Set"(w313) -> ()
                n212 = local write "Gate A Delay"(w316) -> ()
                n213 = local write "Gate B Delay"(w311) -> ()
              }
            }
          }
          event "Update visible/hidden": Value Change {
            n214 = event-data() -> ()  [unwired: 7 out]
            n215 = flat-sequence {
              frame #0 {
                n216 = Not(x="Gate Width: Time / Percent") -> (.not. x?=w330:bool)
                n217 = property on="Gate A % Set" class="DigNum (strict)"("Visible"="Gate Width: Time / Percent") -> ()  [unwired: 2 in, 2 out]
                n218 = property on="Gate B % Set" class="DigNum (strict)"("Visible"="Gate Width: Time / Percent") -> ()  [unwired: 2 in, 2 out]
                n219 = property on="Gate A % Current" class="DigNum (strict)"("Visible"="Gate Width: Time / Percent") -> ()  [unwired: 2 in, 2 out]
                n220 = property on="Gate B % Current" class="DigNum (strict)"("Visible"="Gate Width: Time / Percent") -> ()  [unwired: 2 in, 2 out]
                n221 = property on="Gate B Width Set" class="DigNum (strict)"("Visible"=w330) -> ()  [unwired: 2 in, 2 out]
                n222 = property on="Gate B Width" class="DigNum (strict)"("Visible"=w330) -> ()  [unwired: 2 in, 2 out]
                n223 = property on="Gate A Width" class="DigNum (strict)"("Visible"=w330) -> ()  [unwired: 2 in, 2 out]
                n224 = property on="Gate A Width Set" class="DigNum (strict)"("Visible"=w330) -> ()  [unwired: 2 in, 2 out]
              }
              frame #1 {
                n225 = local read "# Triggers vs Freq/Time"() -> (w332:bool)
                n226 = local read "Internal / External"() -> (w333:bool)
                n227 = Not(x=w332) -> (.not. x?=w334:bool)
                n228 = Not(x=w333) -> (.not. x?=w331:bool)
                n229 = And(x=w333, y=w332) -> (x .and. y?=w336:bool)
                n230 = property on="# Triggers vs Freq/Time" class="Bool (strict)"("Visible"=w333) -> ()  [unwired: 2 in, 2 out]
                n231 = Or(x=w331, y=w332) -> (x .or. y?=w337:bool)
                n232 = And(x=w333, y=w334) -> (x .and. y?=w335:bool)
                n233 = property on="Set Count Time" class="Bool"("Visible"=w331) -> ()  [unwired: 2 in, 2 out]
                n234 = property on="Trigger Freq Set" class="DigNum (strict)"("Visible"=w336) -> ()  [unwired: 2 in, 2 out]
                n235 = property on="Set Time & Freq." class="Bool"("Visible"=w336) -> ()  [unwired: 2 in, 2 out]
                n236 = property on="Trigger Freq Current" class="DigNum (strict)"("Visible"=w336) -> ()  [unwired: 2 in, 2 out]
                n237 = property on="Count Time Current" class="DigNum (strict)"("Visible"=w337) -> ()  [unwired: 2 in, 2 out]
                n238 = property on="Count Time Set" class="DigNum (strict)"("Visible"=w337) -> ()  [unwired: 2 in, 2 out]
                n239 = property on="# of Cycles Set" class="DigNum (strict)"("Visible"=w335) -> ()  [unwired: 2 in, 2 out]
                n240 = property on="# of Cycles Current" class="DigNum (strict)"("Visible"=w335) -> ()  [unwired: 2 in, 2 out]
                n241 = property on="Set # of Triggers" class="Bool"("Visible"=w335) -> ()  [unwired: 2 in, 2 out]
              }
            }
            n242 = local write "Update visible/hidden"(FALSE ("Update visiible/hidden")) -> ()
          }
        }
        n243 = call <vilib>:"Simple Error Handler.vi"("error in (no error)"=w26) -> ("error out"=w25:errorcluster)  [unwired: 1 in, 7 out]
      }
    }
    frame #2 {
    }
  }
  "error out" <- w2
